vi "CreateCopyScriptTest.vi"(8 "error in (no error)":errorcluster, 11 "Test Project Name":string="IOPluginWizardTest") -> (0 "error out":errorcluster, 3 "New Project Location":path)   [LabVIEW 2020]
uses:
  IO PE Creation MDO/ADAS_IO_Template_MDO.lvclass
  C:/Program Files/National Instruments/LabVIEW 2020/resource/dialog/NewProjectWizard/MetaDataObj/MetaDataObj.lvclass
  <vilib>/LabVIEW Icon API/lv_icon/Classes/Icon/Icon.lvclass
  <resource>/dialog/NewProjectWizard/MetaDataObj/MetaDataObj.lvclass/MetaDataObj.ctl
  <resource>/dialog/NewProjectWizard/MetaDataObj/Accessors/Write Project Root.vi
  <resource>/dialog/NewProjectWizard/MetaDataObj/Accessors/Write Project Name.vi
  <resource>/dialog/NewProjectWizard/MetaDataObj/Accessors/Write Overlay Pixmap.vi
  <vilib>/addons/_JKI Toolkits/Caraya/classes/Assert/Assert Not Error.vi
  <vilib>/addons/_JKI Toolkits/Caraya/classes/Assert/Assert True.vi
  <vilib>/addons/_JKI Toolkits/Caraya/classes/Assert/Assert Equal Value_Variant.vi
  <resource>/dialog/NewProjectWizard/Project Copying/NI_NPW_Project Copying.lvlib
  <vilib>/addons/_JKI Toolkits/Caraya/classes/Assert/Assert.lvclass
  <vilib>/addons/_JKI Toolkits/Caraya/classes/Test/Test.lvclass
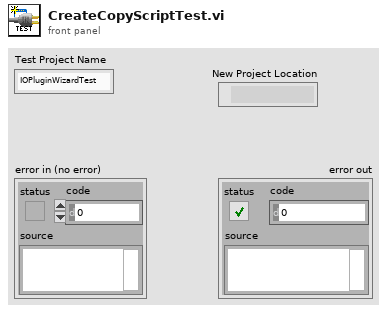
[diagram p1: front panel]
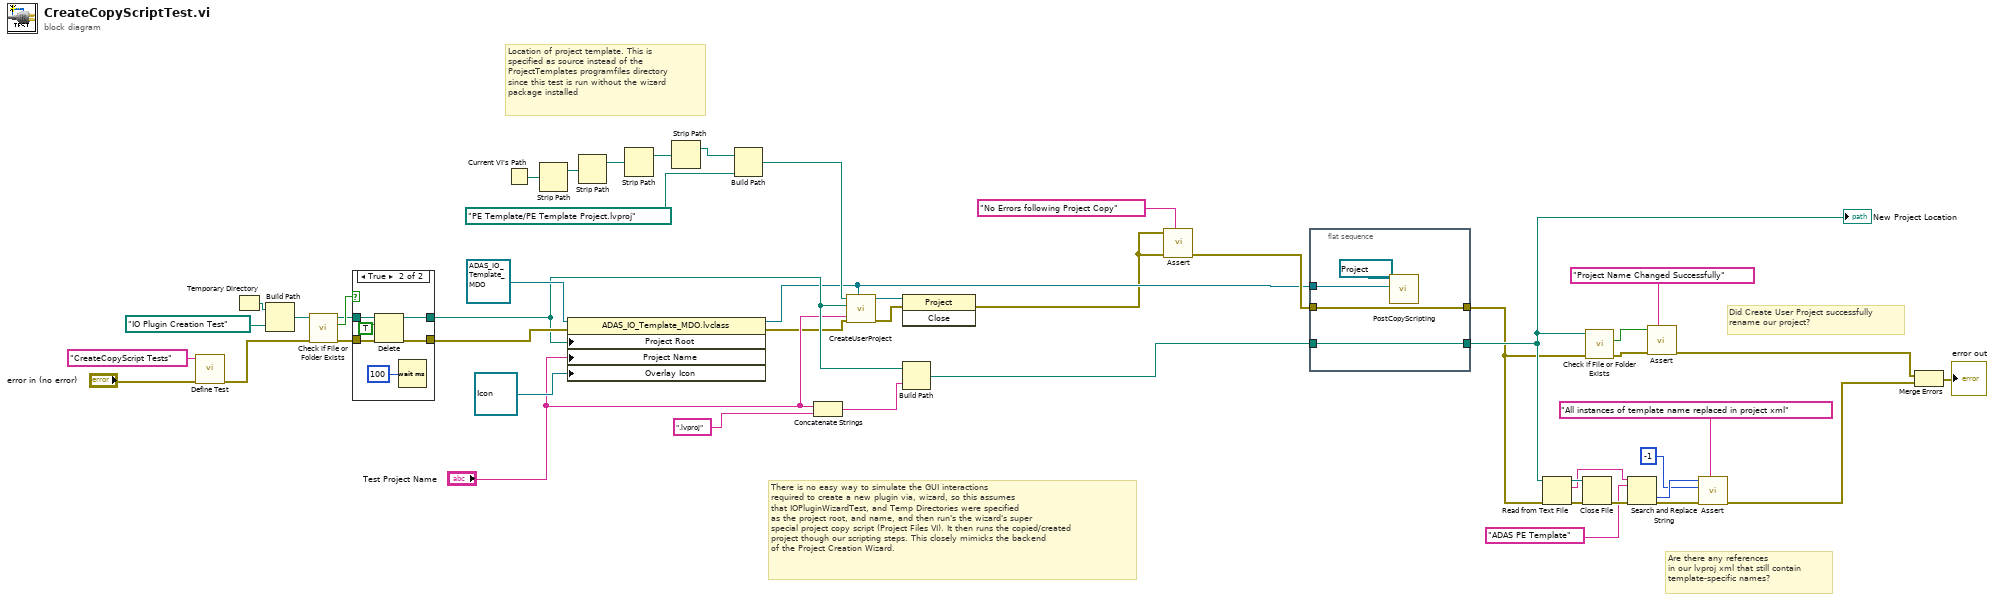
[diagram p0: block diagram]
diagram:
  # "Are there any references \nin our lvproj xml that still contain\ntemplate-specific names?"
  # "Did Create User Project successfully\nrename our project?"
  # "Location of project template. This is\nspecified as source instead of the\nProjectTemplates programfiles directory\nsince this test is run without the wizard\npackage installed"
  # "There is no easy way to simulate the GUI interactions\nrequired to create a new plugin via, wizard, so this assumes\nthat IOPluginWizardTest, and Temp Directories were specified\nas the project root, and name, and then run's the wizard's super\nspecial project copy script (Project Files VI). It then runs the copied/created\nproject though our scripting steps. This closely mimicks the backend\nof the Project Creation Wizard."
  n1 = call <vilib>:"Define Test.vi"("error in (no error)"="error in (no error)", "Label (VI Title)"="CreateCopyScript Tests") -> ("error out"=w3:errorcluster)  [unwired: 9 in]
  n2 = Temporary Directory() -> (w46:path)
  n3 = Build Path(base path=w46, name or relative path=path "IO Plugin Creation Test") -> (appended path=w41:path)
  n4 = call <vilib>:"Check if File or Folder Exists.vi"("error in (no error)"=w3, "path"=w41) -> ("error out"=w38:errorcluster, "file or folder exists?"=w40:bool, "dup path"=w39:path)  [unwired: 7 in]
  n5 = case shown="True" w40 {
    tunnel: w39 -> [w50 w55]
    tunnel: w38 -> [w49 w54]
    tunnel: [w50 w53] -> w33
    tunnel: [w49 w52] -> w35
    frame False {
    }
    frame True {
      n6 = Delete(path (use dialog)=w55, entire hierarchy (F)=TRUE, error in=w54) -> (deleted path=w53:path, error out=w52:errorcluster)  [unwired: 2 in, 1 out]
      n7 = Wait (ms)(milliseconds to wait=u32 100) -> ()  [unwired: 1 out]
    }
  }
  n8 = Current VI's Path() -> (path=w44:path)
  n9 = Strip Path(path=w44) -> (stripped path=w43:path)  [unwired: 1 out]
  n10 = property class="ADAS_IO_Template_MDO.lvclass"(reference=refnum<class "ADAS_IO_Template_MDO.lvclass"> refnum ("ADAS_IO_Template_MDO.lvclass"), error in=w35, "Project Root"=w33, "Project Name"="Test Project Name", "Overlay Icon"=refnum<class "Icon.lvclass"> refnum) -> (reference out=w8:refnum<class "ADAS_IO_Template_MDO.lvclass">, error out=w6:errorcluster)
  n11 = Strip Path(path=w43) -> (stripped path=w48:path)  [unwired: 1 out]
  n12 = Strip Path(path=w48) -> (stripped path=w2:path)  [unwired: 1 out]
  n13 = Strip Path(path=w2) -> (stripped path=w1:path)  [unwired: 1 out]
  n14 = Build Path(base path=w1, name or relative path=path "PE Template/PE Template Project.lvproj") -> (appended path=w36:path)
  n15 = Concatenate Strings("Test Project Name", ".lvproj" ("string")) -> (w20:string)
  n16 = call <resource>:"CreateUserProject.vi"("Target Project Name"="Test Project Name", "MetaDataObj"=w8, "error in (no error)"=w6, "Target Path"=w33, "Source Project Path"=w36) -> ("error out"=w16:errorcluster, "Project"=w17:refnum<vi>)  [unwired: 5 in]
  n17 = invoke class="Project" method="Close"(reference=w17, error in=w16) -> (error out=w7:errorcluster)  [unwired: 1 in, 2 out]
  n18 = Build Path(base path=w33, name or relative path=w20) -> (appended path=w32:path)
  n19 = call-poly <vilib>:"Assert.vi"("Label"="No Errors following Project Copy", "error in (no error)"=w7, "Not Error?"=w7) -> ("error out"=w13:errorcluster)  [unwired: 8 in]
  n20 = flat-sequence {
    tunnel: w8 -> [w60]
    tunnel: w13 -> [w58]
    tunnel: w32 -> [w59]
    tunnel: [w59] -> w19
    tunnel: [w58] -> w15
    frame #0 {
      n21 = call "PostCopyScripting.vi"("MetaDataObj"=w60, "User Project"=refnum<vi> refnum) -> ()  [unwired: 10 in]
    }
  }
  n22 = Read from Text File(file (use dialog)=w19, error in=w15) -> (refnum out=w30:refnum<file>, text=w29:string, error out=w31:errorcluster)  [unwired: 2 in, 1 out]
  n23 = Close File(refnum=w30, error in=w31) -> (error out=w25:errorcluster)  [unwired: 1 out]
  n24 = call <vilib>:"Check if File or Folder Exists.vi"("error in (no error)"=w15, "path"=w19) -> ("error out"=w14:errorcluster, "file or folder exists?"=w18:bool)  [unwired: 7 in, 1 out]
  n25 = Search and Replace String(input string=w29, search string="ADAS PE Template", error in=w25) -> (offset past replacement=w28:i32, error out=w24:errorcluster)  [unwired: 5 in, 2 out]
  n26 = call-poly <vilib>:"Assert.vi"("Label"="Project Name Changed Successfully", "error in (no error)"=w14, "True?"=w18) -> ("error out"=w10:errorcluster)  [unwired: 8 in]
  n27 = call-poly <vilib>:"Assert.vi"("Label"="All instances of template name replaced in project xml", "error in (no error)"=w24, "Y"=-1 ("offset past replacement"), "X"=w28) -> ("error out"=w11:errorcluster)  [unwired: 7 in]
  n28 = Merge Errors(w10, w11) -> (→"error out":errorcluster)
  "New Project Location" <- w19
